vi "Set Scaling.vi"(8 "error in (no error)":errorcluster, 10 "Scaling":cluster{"K":dbl, "N":dbl}[](array[cluster]), 11 "ArduinoAI in":refnum<class "ArduinoAI.lvclass">) -> (0 "error out":errorcluster, 3 "ArduinoAI out":refnum<class "ArduinoAI.lvclass">)   [LabVIEW 2020, in "ArduinoAI.lvclass"]
uses:
  ArduinoAI.lvclass
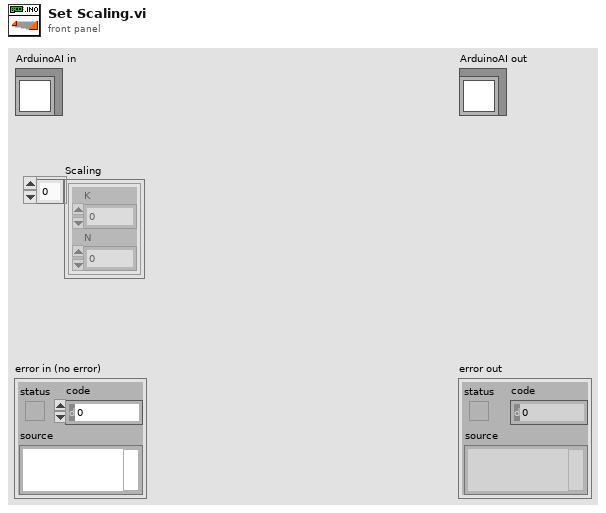
[diagram p1: front panel]
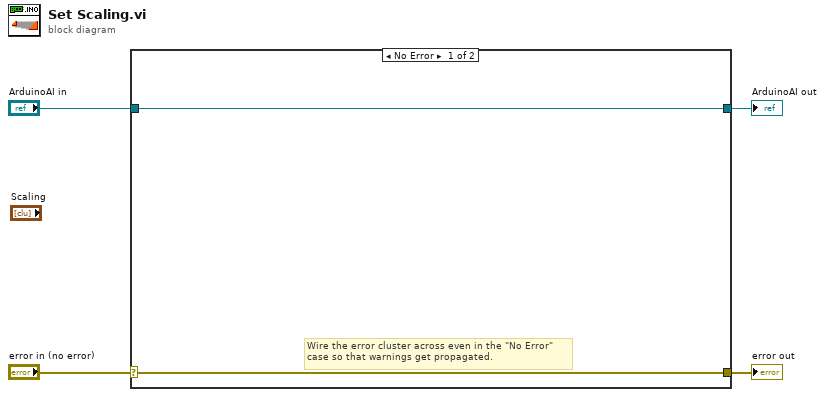
[diagram p0: block diagram]
diagram:
  n1 = case shown="No Error" "error in (no error)" {
    selector: "error in (no error)" -> [w5 w8]
    tunnel: [w5 w8] -> w3
    tunnel: [w6 w7] -> w1
    tunnel: "ArduinoAI in" -> [w6 w7]
    frame No Error {
      # "Wire the error cluster across even in the \"No Error\"\ncase so that warnings get propagated."
    }
    frame Error {
    }
  }
  "error out" <- w3
  "ArduinoAI out" <- w1
